vi "Convert Channel Parameter to Channel and Properties.vi"(10 "channel type":T1, 11 "channel parameter":T3={"name"="", "default value"=0.0, "unit"="", "Parameter"={"start index"=0, "size"=1, "encoding"=enum."BNR", "signed"=FALSE, "scale multiplier"=1.0, "scale offset"=0.0}}) -> (1 "property values":variant[](array[variant]), 2 "property names":string[](array[string]), 3 "channel":T2, 5 "name":string)   [LabVIEW 2020, in "Communication Bus Template Scripting.lvlib"]
doc: "converts channel parameters to channel and properties \n\nNote that channels and properties must be created during configuration. Values for existing properties can be updated after deployment."
uses:
  Communication Bus Template Scripting.lvlib
  <vilib>/NI VeriStand/Custom Device API/Custom Device Channel Type.ctl
  <vilib>/NI VeriStand/Custom Device API/Custom Device API.lvlib
  <vilib>/NI VeriStand/Custom Device API/Custom Device Channel.ctl
  Constants.vi
  Encoding and Decoding/Encoding.ctl
  Encoding and Decoding/Encoding and Decoding.lvlib
  Protocol/Implementations/ARINC429/Parameter Definition.ctl
  Protocol/Implementations/ARINC429/ARINC 429.lvclass
  Git/niveristand-communications-bus-template/Source/Custom Device Support/Shared/VS Channel Definition for Parameter.ctl
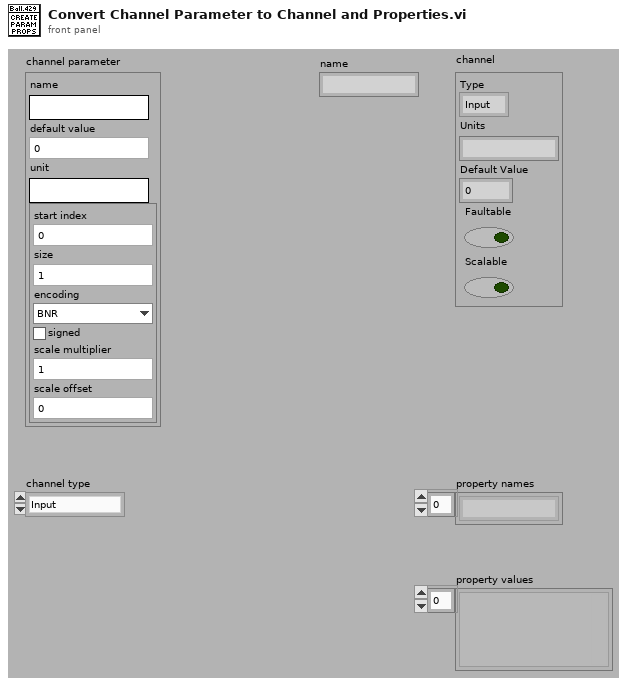
[diagram p1: front panel]
types:
  T1 = typedef "Custom Device API.lvlib/Custom Device Channel Type.ctl" = enum16{"Input", "Output"}
  T2 = typedef "Custom Device API.lvlib/Custom Device Channel.ctl" = cluster{"Type":T1, "Units":string, "Default Value":dbl, "Faultable":bool, "Scalable":bool}
  T3 = typedef "Communication Bus Template Scripting.lvlib/VS Channel Definition for Parameter.ctl" = cluster{"name":string, "default value":dbl, "unit":string, "Parameter":T4}
  T4 = typedef "ARINC 429.lvclass/Parameter Definition.ctl" = cluster{"start index":i32, "size":i32, "encoding":T5, "signed":bool, "scale multiplier":dbl, "scale offset":dbl}
  T5 = typedef "Encoding and Decoding.lvlib/Encoding.ctl" = enum16{"BNR", "BCD", "Discrete"}
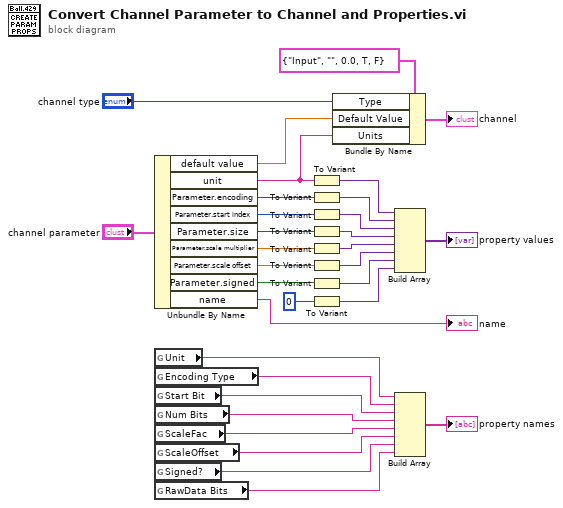
[diagram p0: block diagram]
diagram:
  n1 = Unbundle By Name("channel parameter") -> ("default value"=w4:dbl, "unit"=w3:string, "Parameter.encoding"=w20:T5, "Parameter.start index"=w12:i32, "Parameter.size"=w11:i32, "Parameter.scale multiplier"=w10:dbl, "Parameter.scale offset"=w9:dbl, "Parameter.signed"=w8:bool, "name"=→"name":string)
  n2 = global read "Constants.vi" "Unit"() -> (w7:string)
  n3 = global read "Constants.vi" "Encoding Type"() -> (w19:string)
  n4 = global read "Constants.vi" "Start Bit"() -> (w18:string)
  n5 = global read "Constants.vi" "Num Bits"() -> (w17:string)
  n6 = global read "Constants.vi" "ScaleFac"() -> (w16:string)
  n7 = global read "Constants.vi" "ScaleOffset"() -> (w15:string)
  n8 = global read "Constants.vi" "Signed?"() -> (w14:string)
  n9 = global read "Constants.vi" "RawData Bits"() -> (w13:string)
  n10 = To Variant(anything=w3) -> (Variant=w6:variant)
  n11 = To Variant(anything=w20) -> (Variant=w22:variant)
  n12 = To Variant(anything=w12) -> (Variant=w31:variant)
  n13 = To Variant(anything=w11) -> (Variant=w30:variant)
  n14 = To Variant(anything=w10) -> (Variant=w28:variant)
  n15 = To Variant(anything=w9) -> (Variant=w27:variant)
  n16 = To Variant(anything=w8) -> (Variant=w26:variant)
  n17 = To Variant(anything=u32 0 ("y")) -> (Variant=w25:variant)
  n18 = Bundle By Name(cluster=T2 {"Type"=enum."Input", "Units"="", "Default Value"=0.0, "Faultable"=TRUE, "Scalable"=FALSE} ("Channel"), "Type"="channel type", "Default Value"=w4, "Units"=w3) -> (→"channel":T2)
  n19 = Build Array(w6, w22, w31, w30, w28, w27, w26, w25) -> (→"property values":variant[])
  n20 = Build Array(w7, w19, w18, w17, w16, w15, w14, w13) -> (→"property names":string[])
